vi "basic-dependency-test.vi"(8 "error in (no error)":errorcluster) -> (0 "error out":errorcluster)   [LabVIEW 2013]
uses:
  src/SMO/SMO.lvclass
  src/SMO/Typedefs/SMOState --Enum.ctl
  <vilib>/addons/_JKI Toolkits/Caraya/classes/Test/Test.lvclass
  <vilib>/addons/_JKI Toolkits/Caraya/classes/Assert/Assert.lvclass
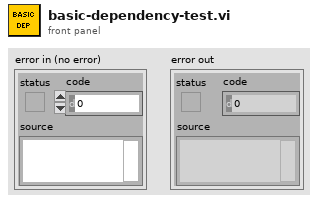
[diagram p1: front panel]
types:
  T1 = typedef "SMO.lvclass/SMOState --Enum.ctl" = enum16{"unknown", "Created", "Started", "Stopped"}
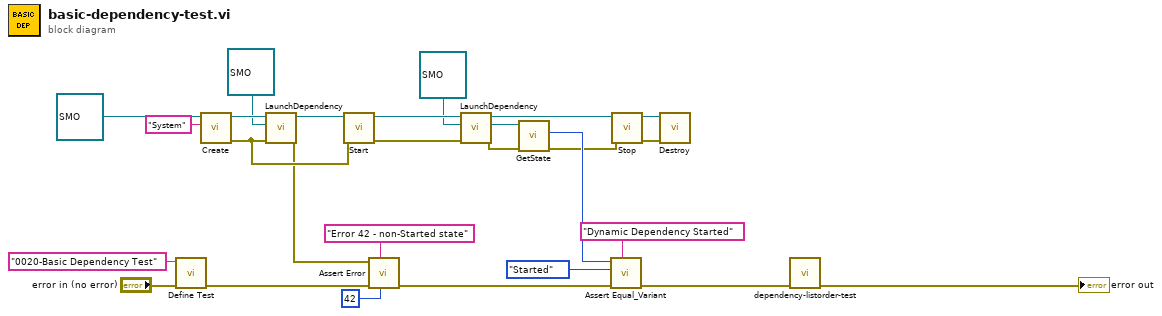
[diagram p0: block diagram]
diagram:
  n1 = call <vilib>:"Define Test.vi"("error in (no error)"="error in (no error)", "Label (VI Title)"="0020-Basic Dependency Test") -> ("error out"=w18:errorcluster)  [unwired: 9 in]
  n2 = call "Create.vi"("Subsystem Name (optional)"="System", "SMO"=refnum<class "SMO.lvclass"> refnum ("SMO.lvclass")) -> ("error out"=w15:errorcluster, "SMO out"=w23:refnum<class "SMO.lvclass">)  [unwired: 7 in, 1 out]
  n3 = call "LaunchDependency.vi"("error in (no error)"=w15, "Dependency Type"=refnum<class "SMO.lvclass"> refnum ("SMO.lvclass"), "SMO in"=w23) -> ("error out"=w14:errorcluster, "SMO out"=w22:refnum<class "SMO.lvclass">)  [unwired: 5 in, 2 out]
  n4 = call "Start.vi"("error in (no error)"=w15, "SMO"=w22) -> ("error out"=w12:errorcluster, "SMO out"=w13:refnum<class "SMO.lvclass">)  [unwired: 8 in]
  n5 = call <vilib>:"Assert Error.vi"("error code (1)"=42, "Label"="Error 42 - non-Started state", "error in (no error)"=w18, "Error?"=w14) -> ("error out"=w7:errorcluster)  [unwired: 7 in]
  n6 = call "LaunchDependency.vi"("error in (no error)"=w12, "Dependency Type"=refnum<class "SMO.lvclass"> refnum ("SMO.lvclass"), "SMO in"=w13) -> ("error out"=w8:errorcluster, "Dependency Reference"=w9:refnum<class "SMO.lvclass">, "SMO out"=w10:refnum<class "SMO.lvclass">)  [unwired: 5 in, 1 out]
  n7 = call "GetState.vi"("error in (no error)"=w8, "SMO"=w9) -> ("error out"=w3:errorcluster, "SMO State"=w6:T1)  [unwired: 7 in, 1 out]
  n8 = call <vilib>:"Assert Equal_Variant.vi"("Label"="Dynamic Dependency Started", "error in (no error)"=w7, "Y"=SMOState_--Enum."Started" ("SMO State"), "X"=w6) -> ("error out"=w2:errorcluster)  [unwired: 7 in]
  n9 = call "Stop.vi"("error in (no error)"=w3, "SMO"=w10) -> ("error out"=w20:errorcluster, "SMO out"=w19:refnum<class "SMO.lvclass">)  [unwired: 8 in]
  n10 = call "Destroy.vi"("error in (no error)"=w20, "SMO"=w19) -> ()  [unwired: 9 in, 1 out]
  n11 = call "dependency-listorder-test.vi"("error in (no error)"=w2) -> ("error out"=→"error out":errorcluster)  [unwired: 10 in]
